vi "Set Velocity.vi"(1 "Axis":string, 2 "Voltage":dbl) -> (0 "Command":string)   [LabVIEW 2011]
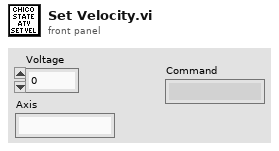
[diagram p1: front panel]
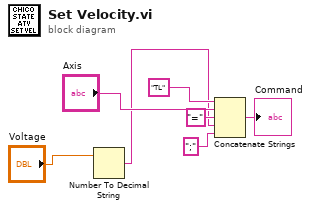
[diagram p0: block diagram]
diagram:
  n1 = Number To Decimal String(number="Voltage") -> (decimal integer string=w1:string)  [unwired: 1 in]
  n2 = Concatenate Strings("TL" ("string"), "Axis", "=" ("string"), w1, ";" ("string")) -> (→"Command":string)
